vi "_TCP-IP Mgr.Test.vi"() -> ()   [LabVIEW 2024, in "EQMF.lvlib" / "TCP-IP.lvlib"]
uses:
  TCP-IP.lvlib
  TCP-IP Mgr.Cluster - Q Message Templates.ctl
  Queues/Q.Element.ctl
  TCP-IP Mgr.Config.ctl
  Queues/Queue Utils.lvlib
panel:
  in  "Tab Control":enum32{"Config", "Operate"}(tab)
  in  "C Config":T1={"IP"="127.0.0.1", "Port"=8500, "Listener"=FALSE, "Enable"=TRUE}
  in  "Status_Rcv Q Client":T2={"Status.Q.Msg"={"Cmd"="Task", "Sub"="Client Status", "Data1"=variant, "Data2"=variant}, "Rcv.Q.Msg"={"Cmd"="Task", "Sub"="Client Rcv", "Data1"=variant, "Data2"=variant}}
  in  "Status_Rcv Q Listener":T2={"Status.Q.Msg"={"Cmd"="Task", "Sub"="Listener Status", "Data1"=variant, "Data2"=variant}, "Rcv.Q.Msg"={"Cmd"="Task", "Sub"="Listener Rcv", "Data1"=variant, "Data2"=variant}}
  in  "L Config":T1={"IP"="127.0.0.1", "Port"=8500, "Listener"=TRUE, "Enable"=TRUE}
  in  "Client Disconnect":bool
  in  "C Show":bool
  in  "L Show":bool
  in  "L Clear":bool
  in  "C Clear":bool
  out "C Status":bool
  out "L Status":bool
  in  "L Send":bool
  in  "C Send":bool
  in  "Client Connect":bool
  out "Client Data":string
  out "Listener Data":string
  in  "Listener Data Out":string
  in  "Client Data Out":string
  out "error out":errorcluster
  in  "Exit":bool
  # "Listener"
  # "Client"
  # "Listener"
  # "Client"
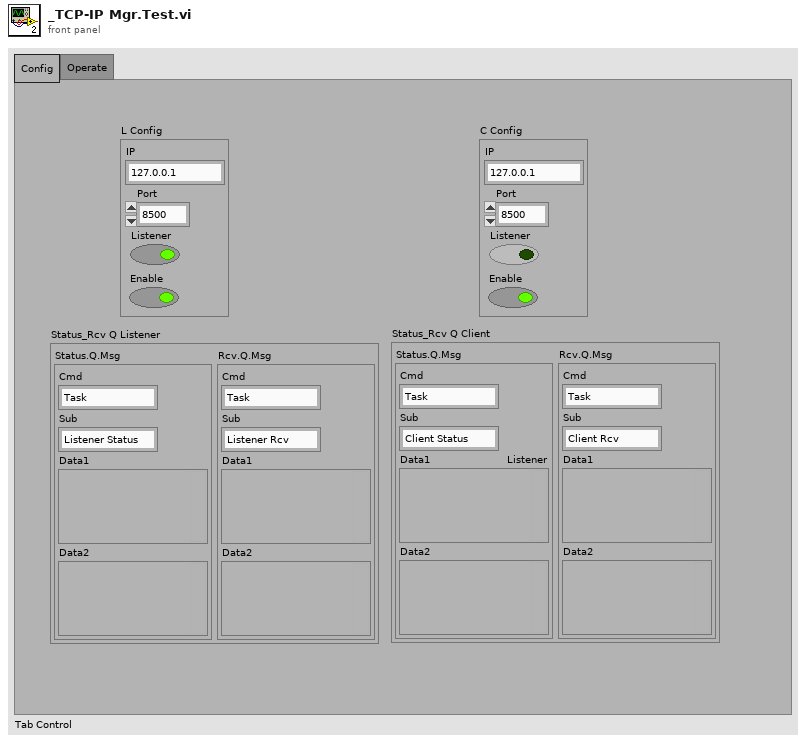
[diagram p1: front panel]
types:
  T1 = typedef "EQMF.lvlib/TCP-IP.lvlib/TCP-IP Mgr.Config.ctl" = cluster{"IP":string, "Port":u16, "Listener":bool, "Enable":bool}
  T2 = typedef "EQMF.lvlib/TCP-IP.lvlib/TCP-IP Mgr.Cluster - Q Message Templates.ctl" = cluster{"Status.Q.Msg":T3, "Rcv.Q.Msg":T3}
  T3 = typedef "EQMF.lvlib/Queue Utils.lvlib/Q.Element.ctl" = cluster{"Cmd":string, "Sub":string, "Data1":variant, "Data2":variant}
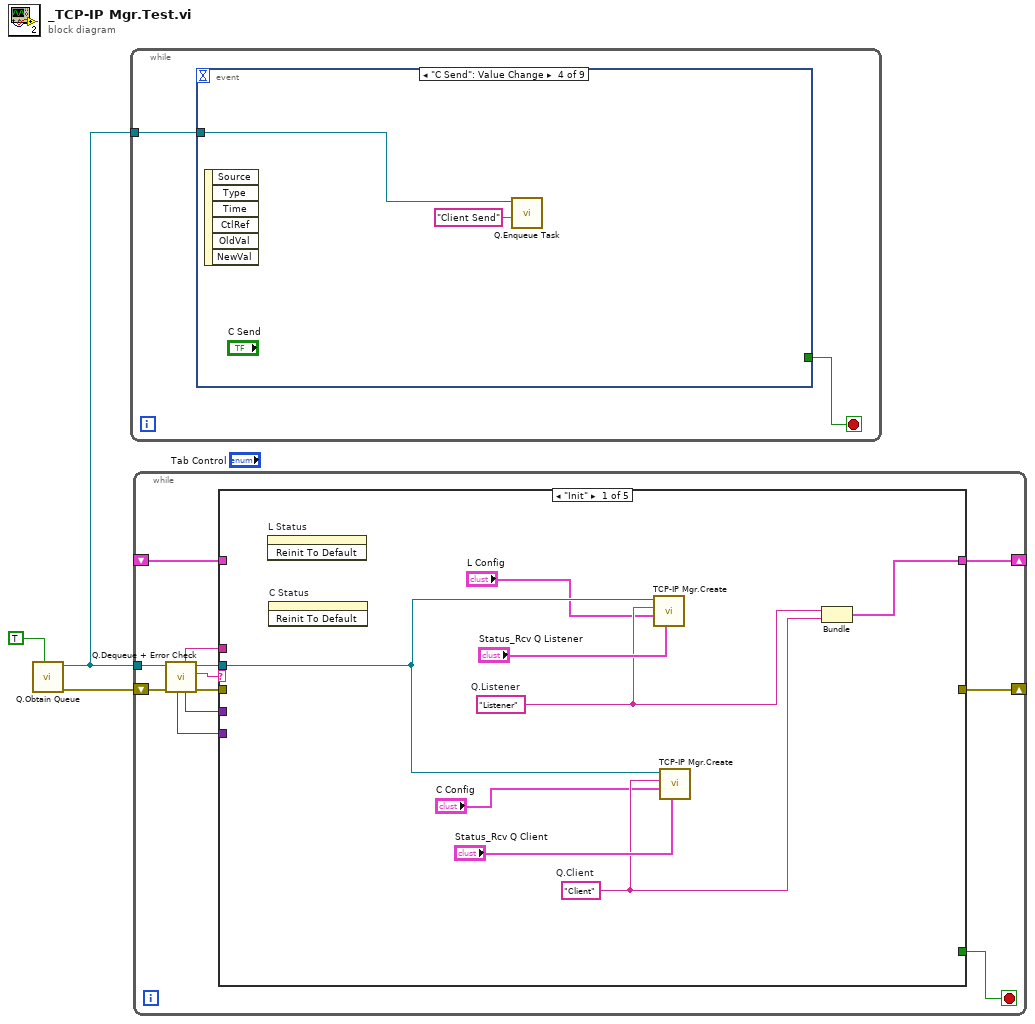
[diagram p0: block diagram]
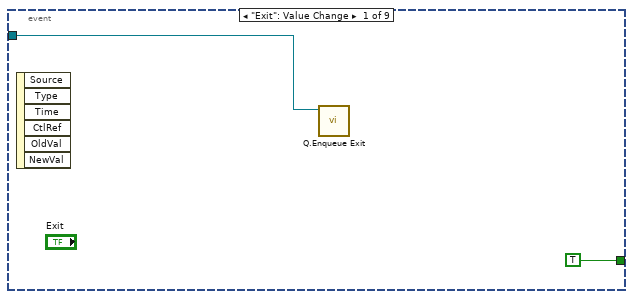
[diagram p2: hidden frame]
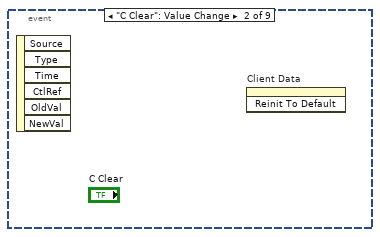
[diagram p3: hidden frame]
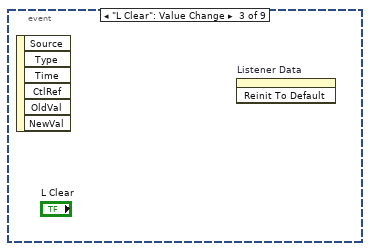
[diagram p4: hidden frame]
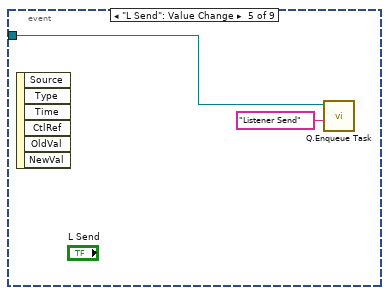
[diagram p5: hidden frame]
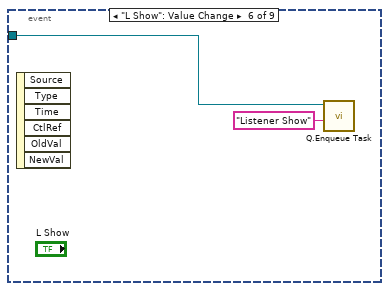
[diagram p6: hidden frame]
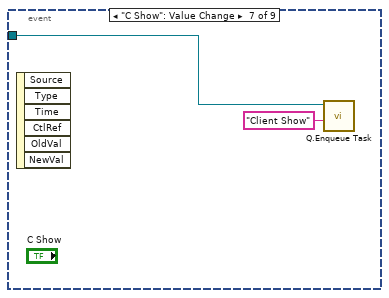
[diagram p7: hidden frame]
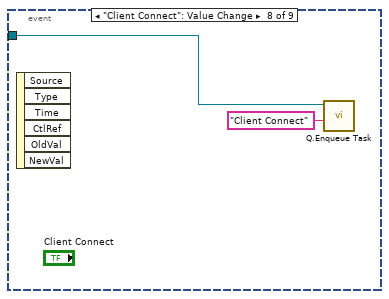
[diagram p8: hidden frame]
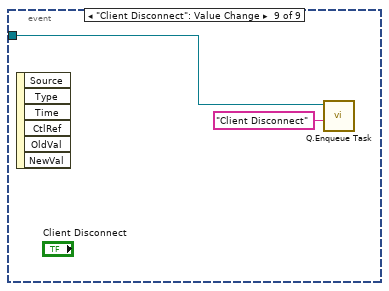
[diagram p9: hidden frame]
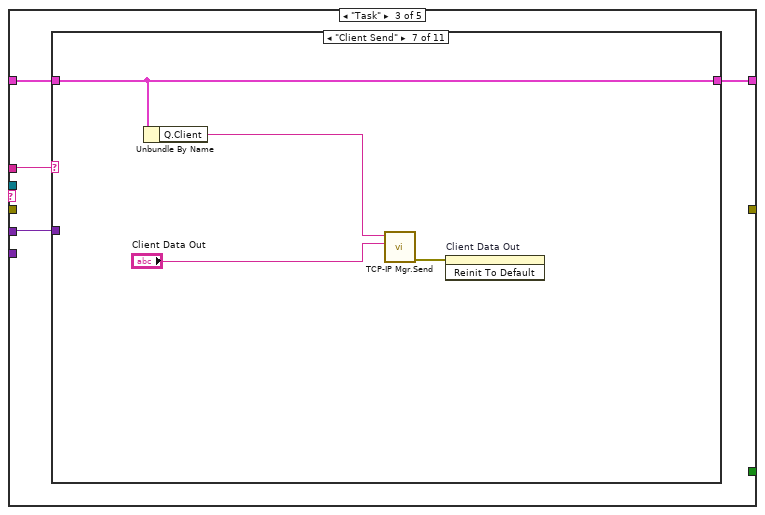
[diagram p11: hidden frame]
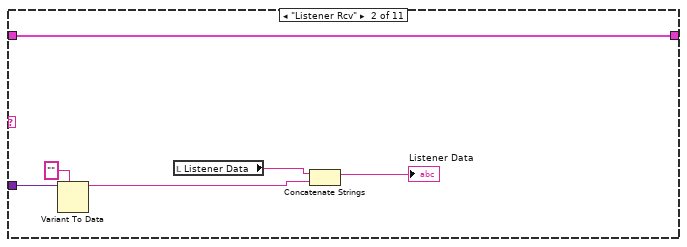
[diagram p13: hidden frame]
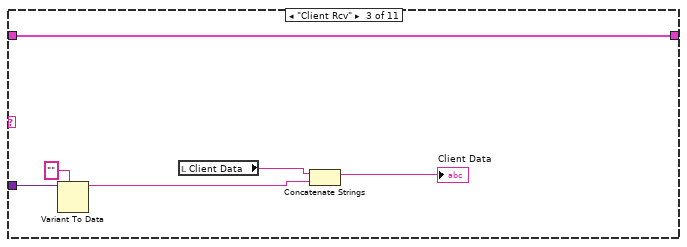
[diagram p14: hidden frame]
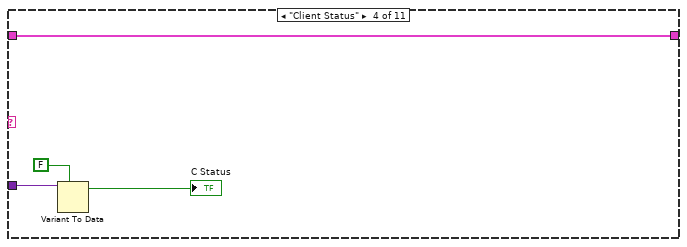
[diagram p15: hidden frame]
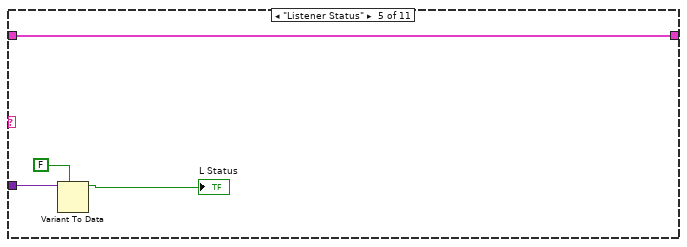
[diagram p16: hidden frame]
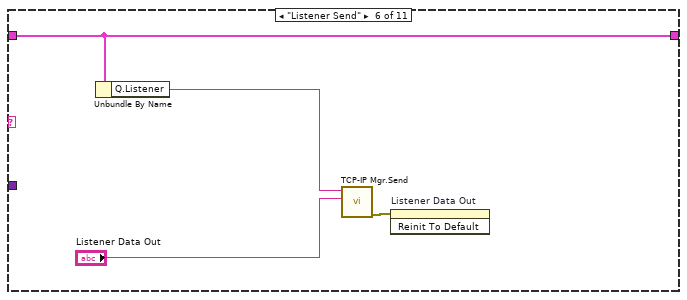
[diagram p17: hidden frame]
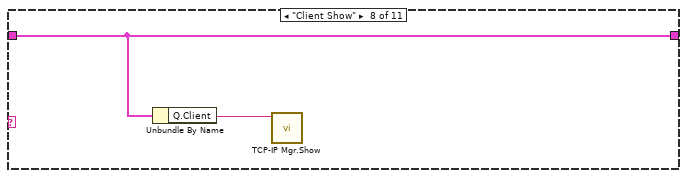
[diagram p18: hidden frame]
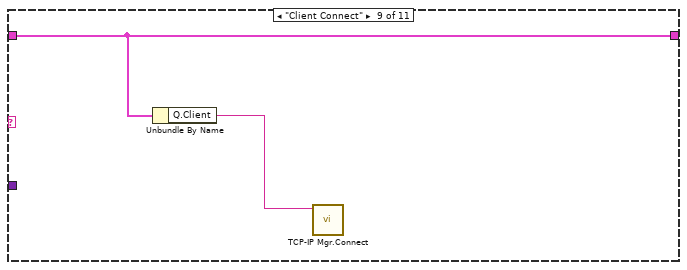
[diagram p19: hidden frame]
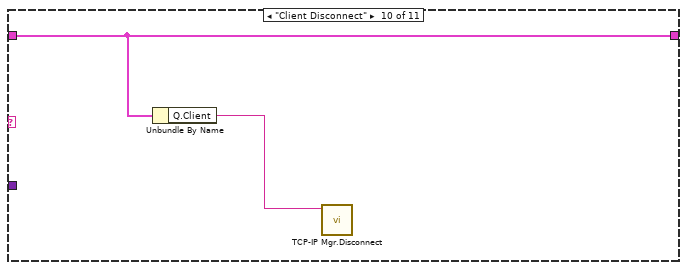
[diagram p20: hidden frame]
diagram:
  n1 = call "Q.Obtain Queue.vi"("Enqueue Init"=TRUE) -> ("error out"=w2:errorcluster, "Q Out"=w3:refnum<queue>)  [unwired: 8 in, 1 out]
  n2 = while {
    tunnel: w3 -> [w5]
    stop <- w4 stop-if-true
    n3 = event shown="[3] \"C Send\": Value Change" {
      selector: _ -> [_ _ _ _ _ _ _ _ _]
      dyn-events: _ -> [_ _ _ _ _ _ _ _ _]
      timeout: _ -> [_ _ _ _ _ _ _ _ _]
      tunnel: w5 -> [w7 _ _ w9 w11 w13 w15 w17 w19]
      tunnel: [TRUE _ _ _ _ _ _ _ _] -> w4
      event "Exit": Value Change {
        n4 = event-data() -> ()  [unwired: 1 in, 6 out]
        n5 = call "Q.Enqueue Exit.vi"("Q In"=w7) -> ()  [unwired: 9 in, 2 out]
      }
      event "C Clear": Value Change {
        n6 = event-data() -> ()  [unwired: 1 in, 6 out]
        n7 = invoke on="Client Data" class="Str" method="Reinit To Default"() -> ()  [unwired: 3 in, 3 out]
      }
      event "L Clear": Value Change {
        n8 = event-data() -> ()  [unwired: 1 in, 6 out]
        n9 = invoke on="Listener Data" class="Str" method="Reinit To Default"() -> ()  [unwired: 3 in, 3 out]
      }
      event "C Send": Value Change {
        n10 = event-data() -> ()  [unwired: 1 in, 6 out]
        n11 = call "Q.Enqueue Task.vi"("Task Name"="Client Send", "Q In"=w9) -> ()  [unwired: 8 in, 2 out]
      }
      event "L Send": Value Change {
        n12 = event-data() -> ()  [unwired: 1 in, 6 out]
        n13 = call "Q.Enqueue Task.vi"("Task Name"="Listener Send", "Q In"=w11) -> ()  [unwired: 8 in, 2 out]
      }
      event "L Show": Value Change {
        n14 = event-data() -> ()  [unwired: 1 in, 6 out]
        n15 = call "Q.Enqueue Task.vi"("Task Name"="Listener Show", "Q In"=w13) -> ()  [unwired: 8 in, 2 out]
      }
      event "C Show": Value Change {
        n16 = event-data() -> ()  [unwired: 1 in, 6 out]
        n17 = call "Q.Enqueue Task.vi"("Task Name"="Client Show", "Q In"=w15) -> ()  [unwired: 8 in, 2 out]
      }
      event "Client Connect": Value Change {
        n18 = event-data() -> ()  [unwired: 1 in, 6 out]
        n19 = call "Q.Enqueue Task.vi"("Task Name"="Client Connect", "Q In"=w17) -> ()  [unwired: 8 in, 2 out]
      }
      event "Client Disconnect": Value Change {
        n20 = event-data() -> ()  [unwired: 1 in, 6 out]
        n21 = call "Q.Enqueue Task.vi"("Task Name"="Client Disconnect", "Q In"=w19) -> ()  [unwired: 8 in, 2 out]
      }
    }
  }
  n22 = while {
    tunnel: w3 -> [w31]
    shift-right: [w23] -> _
    shift-left: w2 -> [w30]
    shift-right: [w20] -> _
    shift-left: _ -> [w21]
    stop <- w22 stop-if-true
    n23 = call "Q.Dequeue + Error Check.vi"("Error In"=w30, "Q In"=w31) -> ("error out"=w28:errorcluster, "Cmd"=w29:string, "Q Out"=w27:refnum<queue>, "Data1"=w25:variant, "Sub"=w26:string, "Data2"=w24:variant)  [unwired: 4 in]
    n24 = case shown="\"Init\"" w29 {
      tunnel: w28 -> [_ _ _ w85 _]
      tunnel: w27 -> [w37 _ _ _ _]
      tunnel: w26 -> [_ _ w44 w87 _]
      tunnel: w25 -> [_ _ w41 w86 _]
      tunnel: w24 -> [_ _ _ _ _]
      tunnel: [_ _ _ errorcluster {"status"=FALSE, "code"=0, "source"=""} ("error constant") _] -> w23
      tunnel: [_ _ _ _ TRUE] -> w22
      tunnel: w21 -> [_ w40 w43 w82 w97]
      tunnel: [w35 w40 w42 w82 w97] -> w20
      frame "Init" {
        w36 = "Client"  # Q.Client
        w34 = "Listener"  # Q.Listener
        n25 = invoke on="L Status" class="Bool (strict)" method="Reinit To Default"() -> ()  [unwired: 3 in, 3 out]
        n26 = invoke on="C Status" class="Bool (strict)" method="Reinit To Default"() -> ()  [unwired: 3 in, 3 out]
        n27 = call "TCP-IP Mgr.Create.vi"("Status_Rcv Q Items"="Status_Rcv Q Listener", "Config"="L Config", "Q Name"=w34, "Parent Q"=w37) -> ()  [unwired: 5 in, 3 out]
        n28 = call "TCP-IP Mgr.Create.vi"("Status_Rcv Q Items"="Status_Rcv Q Client", "Config"="C Config", "Q Name"=w36, "Parent Q"=w37) -> ()  [unwired: 5 in, 3 out]
        n29 = Bundle("Q.Listener"=w34, "Q.Client"=w36) -> (w35:cluster{"Q.Listener":string, "Q.Client":string})  [unwired: 1 in]
      }
      frame "Reset" {
      }
      frame "Task" {
        n30 = case shown="\"Client Send\"" w44 {
          tunnel: w43 -> [w45 w51 w57 w61 w65 w69 w73 w75 w77 w79 w81]
          tunnel: [w45 w51 w57 w61 w65 w69 w73 w75 w77 w79 w81] -> w42
          tunnel: w41 -> [_ w48 w55 w60 w64 _ _ _ _ _ _]
          frame "False", Default {
          }
          frame "Listener Rcv" {
            n31 = Variant To Data(type="", Variant=w48) -> (data=w46:string)  [unwired: 1 in, 1 out]
            n32 = local read "Listener Data"() -> (w50:string)
            n33 = Concatenate Strings(w50, w46) -> (→"Listener Data":string)
          }
          frame "Client Rcv" {
            n34 = Variant To Data(type="", Variant=w55) -> (data=w53:string)  [unwired: 1 in, 1 out]
            n35 = local read "Client Data"() -> (w56:string)
            n36 = Concatenate Strings(w56, w53) -> (→"Client Data":string)
          }
          frame "Client Status" {
            n37 = Variant To Data(type=FALSE, Variant=w60) -> (data=→"C Status":bool)  [unwired: 1 in, 1 out]
          }
          frame "Listener Status" {
            n38 = Variant To Data(type=FALSE, Variant=w64) -> (data=→"L Status":bool)  [unwired: 1 in, 1 out]
          }
          frame "Listener Send" {
            n39 = Unbundle By Name(w69) -> ("Q.Listener"=w68:string)
            n40 = call "TCP-IP Mgr.Send.vi"("Send Data"="Listener Data Out", "Q Name"=w68) -> ("error out"=w66:errorcluster)  [unwired: 9 in]
            n41 = invoke on="Listener Data Out" class="Str" method="Reinit To Default"(error in=w66) -> ()  [unwired: 2 in, 3 out]
          }
          frame "Client Send" {
            n42 = Unbundle By Name(w73) -> ("Q.Client"=w72:string)
            n43 = call "TCP-IP Mgr.Send.vi"("Send Data"="Client Data Out", "Q Name"=w72) -> ("error out"=w71:errorcluster)  [unwired: 9 in]
            n44 = invoke on="Client Data Out" class="Str" method="Reinit To Default"(error in=w71) -> ()  [unwired: 2 in, 3 out]
          }
          frame "Client Show" {
            n45 = Unbundle By Name(w75) -> ("Q.Client"=w74:string)
            n46 = call "TCP-IP Mgr.Show.vi"("Q Name"=w74) -> ()  [unwired: 10 in, 1 out]
          }
          frame "Client Connect" {
            n47 = Unbundle By Name(w77) -> ("Q.Client"=w76:string)
            n48 = call "TCP-IP Mgr.Connect.vi"("Q Name"=w76) -> ()  [unwired: 10 in, 1 out]
          }
          frame "Client Disconnect" {
            n49 = Unbundle By Name(w79) -> ("Q.Client"=w78:string)
            n50 = call "TCP-IP Mgr.Disconnect.vi"("Q Name"=w78) -> ()  [unwired: 10 in, 1 out]
          }
          frame "Listener Show" {
            n51 = Unbundle By Name(w81) -> ("Q.Listener"=w80:string)
            n52 = call "TCP-IP Mgr.Show.vi"("Q Name"=w80) -> ()  [unwired: 10 in, 1 out]
          }
        }
      }
      frame "Error", Default {
        n53 = case shown="\"Error\"" w87 {
          tunnel: w86 -> [_ w91]
          tunnel: w85 -> [w88 _]
          tunnel: [w88 w89] -> w84
          frame Default {
          }
          frame "Error" {
            n54 = Variant To Data(type=errorcluster {"status"=FALSE, "code"=0, "source"=""} ("error out"), Variant=w91) -> (data=w89:errorcluster)  [unwired: 1 in, 1 out]
          }
        }
        "error out" <- w84
      }
      frame "Exit" {
        n55 = Unbundle By Name(w97) -> ("Q.Listener"=w96:string, "Q.Client"=w95:string)
        n56 = call "TCP-IP Mgr.Destroy.vi"("Q Name"=w95) -> ("error out"=w93:errorcluster)  [unwired: 10 in]
        n57 = call <vilib>:"Clear Errors.vi"("error in (no error)"=w93) -> ("error out"=w94:errorcluster)  [unwired: 5 in, 1 out]
        n58 = call "TCP-IP Mgr.Destroy.vi"("error in (no error)"=w94, "Q Name"=w96) -> ("error out"=w92:errorcluster)  [unwired: 9 in]
        n59 = call <vilib>:"Clear Errors.vi"("error in (no error)"=w92) -> ()  [unwired: 5 in, 2 out]
      }
    }
  }
